vi "ep_Filter Specificaiton Conversion.vi"(7 "filter type":T1, 8 "error in (no error)":errorcluster, 10 "ripple specs":T2={"passband"=0.1, "stopband"=40.0, "dB/linear? (T: dB)"=TRUE}, 11 "freq specs [Hz]":T3) -> (0 "error out":errorcluster, 1 "low cutoff freq: fl":dbl, 2 "high cutoff freq: fh":dbl, 3 "min transition band":dbl, 4 "A stop (dB)":dbl format="%.2f")   [LabVIEW 2012, in "NI_EP_Resample_Host.lvlib"]
uses:
  <vilib>/addons/Electrical Power/PQ/Resampling/NI_EP_Resample_Host.lvlib
  <vilib>/Analysis/3filter.llb/Filter Passband Type.ctl
  <vilib>/Analysis/NI_AALBase.lvlib
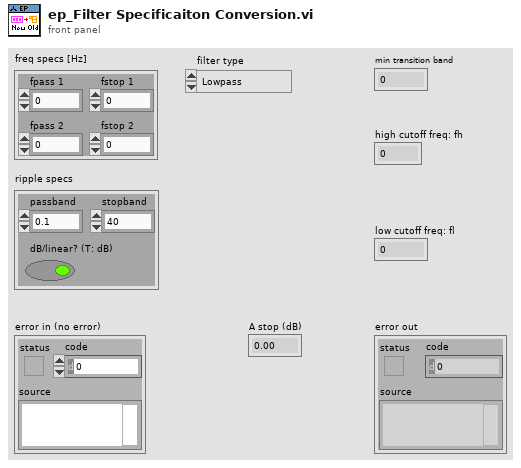
[diagram p1: front panel]
types:
  T1 = typedef "NI_AALBase.lvlib/Filter Passband Type.ctl" = enum32{"Lowpass", "Highpass", "Bandpass", "Bandstop"}
  T2 = cluster{"passband":dbl, "stopband":dbl, "dB/linear? (T: dB)":bool}
  T3 = cluster{"fpass 1":dbl, "fstop 1":dbl, "fpass 2 ":dbl, "fstop 2":dbl}
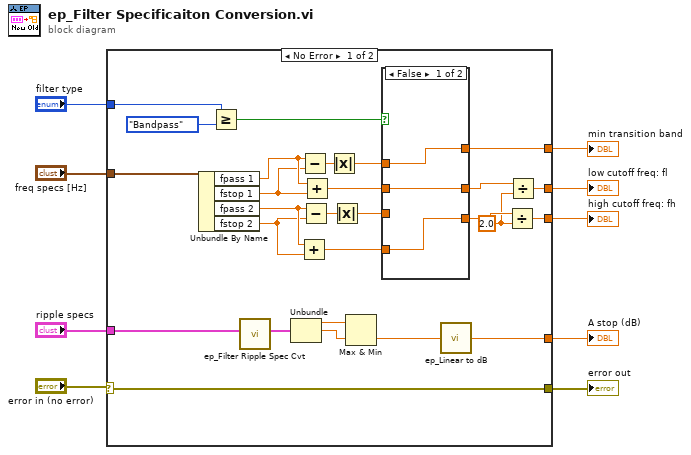
[diagram p0: block diagram]
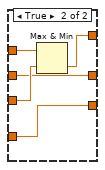
[diagram p2: hidden frame]
diagram:
  n1 = case shown="No Error" "error in (no error)" {
    selector: "error in (no error)" -> [w18 w45]
    tunnel: "freq specs [Hz]" -> [w36 _]
    tunnel: "filter type" -> [w34 _]
    tunnel: [w30 _] -> w8
    tunnel: "ripple specs" -> [w19 _]
    tunnel: [w11 _] -> w6
    tunnel: [w18 w45] -> w4
    tunnel: [w15 _] -> w3
    tunnel: [w14 _] -> w2
    frame No Error {
      w13 = 2.0 ("y")
      n2 = Unbundle By Name(w36) -> ("fpass 1"=w28:dbl, "fstop 1"=w27:dbl, "fpass 2"=w26:dbl, "fstop 2"=w25:dbl)
      n3 = Greater Or Equal?(x=w34, y=Filter_Passband_Type."Bandpass" ("filter type")) -> (x >= y?=w33:bool)
      n4 = call <vilib>:"ep_Filter Ripple Spec Cvt.vi"("ripple specs"=w19) -> ("ripple specs (linear)"=w20:T2)  [unwired: 9 in, 1 out]
      n5 = Unbundle(w20) -> ("passband"=w22:dbl, "stopband"=w21:dbl)  [unwired: 1 out]
      n6 = Add(x=w26, y=w25) -> (x+y=w23:dbl)
      n7 = Subtract(x=w28, y=w27) -> (x-y=w35:dbl)
      n8 = Subtract(x=w26, y=w25) -> (x-y=w29:dbl)
      n9 = Add(x=w28, y=w27) -> (x+y=w24:dbl)
      n10 = Absolute Value(x=w35) -> (abs(x)=w32:dbl)
      n11 = Absolute Value(x=w29) -> (abs(x)=w31:dbl)
      n12 = Max & Min(x=w22, y=w21) -> (min(x,y)=w12:dbl)  [unwired: 1 out]
      n13 = case shown="False" w33 {
        tunnel: w32 -> [w39 w44]
        tunnel: w31 -> [_ w43]
        tunnel: [w39 w42] -> w30
        tunnel: w24 -> [w38 w40]
        tunnel: w23 -> [w37 w41]
        tunnel: [w37 w41] -> w16
        tunnel: [w38 w40] -> w17
        frame False {
        }
        frame True {
          n14 = Max & Min(x=w44, y=w43) -> (min(x,y)=w42:dbl)  [unwired: 1 out]
        }
      }
      n15 = call <vilib>:"ep_Linear to dB.vi"("linear value"=w12) -> ("dB value"=w11:dbl)  [unwired: 1 in]
      n16 = Divide(x=w16, y=w13) -> (x/y=w14:dbl)
      n17 = Divide(x=w17, y=w13) -> (x/y=w15:dbl)
    }
    frame Error {
    }
  }
  "min transition band" <- w8
  "A stop (dB)" <- w6
  "error out" <- w4
  "low cutoff freq: fl" <- w3
  "high cutoff freq: fh" <- w2
